vi "functional global VI.vi"(10 "Enum":T1(ring), 11 "Numeric":dbl) -> (2 "Numeric 2":dbl)   [LabVIEW 2012]
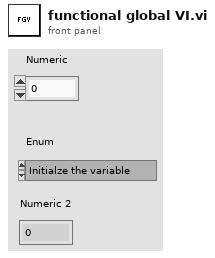
[diagram p1: front panel]
types:
  T1 = enum16{"Initialze the variable", "Increment", "Decrement"}
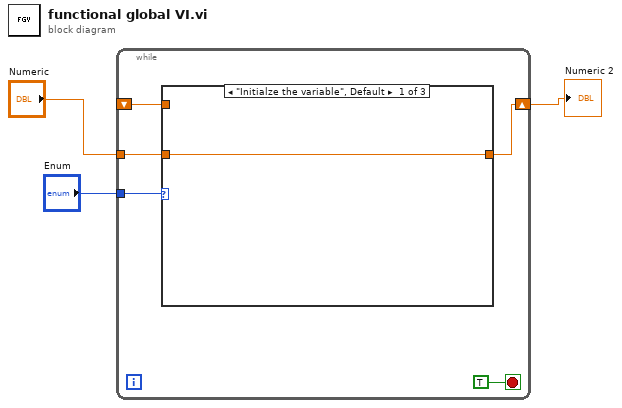
[diagram p0: block diagram]
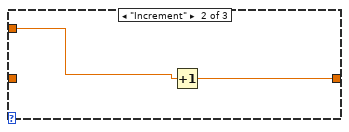
[diagram p2: hidden frame]
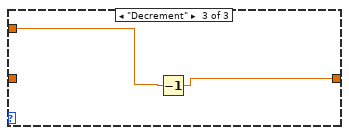
[diagram p3: hidden frame]
diagram:
  n1 = while {
    shift-right: [w7] -> w1
    shift-left: _ -> [w5]
    tunnel: "Enum" -> [w8]
    tunnel: "Numeric" -> [w6]
    stop <- TRUE stop-if-true
    n2 = case shown="\"Initialze the variable\", Default" w8 {
      tunnel: [w9 w11 w13] -> w7
      tunnel: w6 -> [w9 _ _]
      tunnel: w5 -> [_ w10 w12]
      frame "Initialze the variable", Default {
      }
      frame "Increment" {
        n3 = Increment(x=w10) -> (x+1=w11:dbl)
      }
      frame "Decrement" {
        n4 = Decrement(x=w12) -> (x-1=w13:dbl)
      }
    }
  }
  "Numeric 2" <- w1
